vi "SMC_calibrate.vi"(8 "error in (no error)":errorcluster) -> (0 "error out":errorcluster)   [LabVIEW 2015]
uses:
  SMC_SubVIs.llb/SMC_ManagerMode.ctl
  SMC_SubVIs.llb/glb_stop.vi
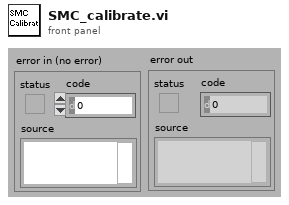
[diagram p1: front panel]
types:
  T1 = typedef "SMC_ManagerMode.ctl" = enum16{"Init", "Get", "SetPosition", "SetStatus", "SetMoving", "SetControllerNr"}
  T2 = typedef "SMC Paras.ctl" = cluster{"VENUS Language":T3, "Number of Axis":u8, "Controller Nr":u8, "Simulation":bool}
  T3 = typedef "VENUSNr.ctl" = enum16{"VENUS 2", "VENUS 1"}
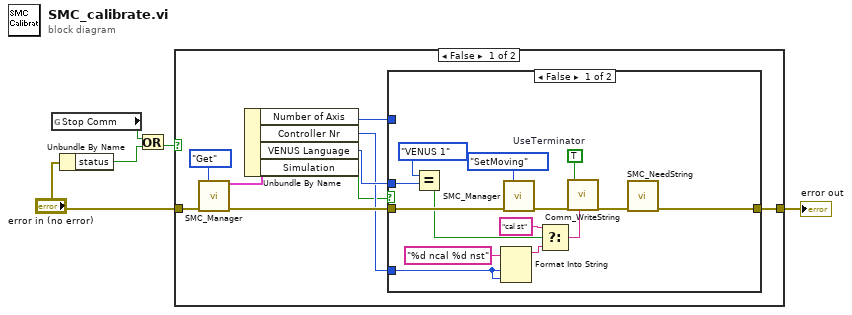
[diagram p0: block diagram]
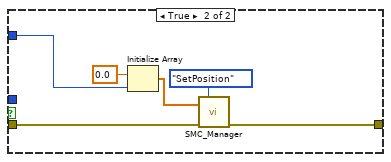
[diagram p2: hidden frame]
diagram:
  n1 = global read "glb_stop.vi" "Stop Comm"() -> (w3:bool)
  n2 = Unbundle By Name("error in (no error)") -> ("status"=w2:bool)
  n3 = Or(x=w3, y=w2) -> (x .or. y?=w1:bool)
  n4 = case shown="False" w1 {
    tunnel: "error in (no error)" -> [w11 w35]
    tunnel: [w14 w35] -> w4
    frame False {
      n5 = call "SMC_Manager.vi"("Mode"=SMC_ManagerMode."Get", "error in (no error)"=w11) -> ("SMC Parameter Out"=w10:T2, "error out"=w12:errorcluster)  [unwired: 9 in, 3 out]
      n6 = Unbundle By Name(w10) -> ("Number of Axis"=w7:u8, "Controller Nr"=w8:u8, "VENUS Language"=w9:T3, "Simulation"=w6:bool)
      n7 = case shown="False" w6 {
        tunnel: w12 -> [w28 w33]
        tunnel: [w25 w32] -> w14
        tunnel: w9 -> [w23 _]
        tunnel: w8 -> [w16 _]
        tunnel: w7 -> [_ w29]
        frame False {
          w15 = TRUE  # UseTerminator
          n8 = Equal?(x=enum16{"VENUS 2", "VENUS 1"}."VENUS 1", y=w23) -> (x = y?=w21:bool)
          n9 = Format Into String(format string="%d ncal %d nst" ("Format String"), w16, w16) -> (resulting string=w18:string)  [unwired: 2 in, 1 out]
          n10 = call "SMC_Manager.vi"("Mode"=SMC_ManagerMode."SetMoving", "error in (no error)"=w28) -> ("error out"=w24:errorcluster)  [unwired: 9 in, 4 out]
          n11 = Select(t="cal st" ("Substring"), s=w21, f=w18) -> (s? t:f=w20:string)
          n12 = call "Comm_WriteString.vi"("string to write"=w20, "error in (no error)"=w24, "UseTerminator"=w15) -> ("error out"=w26:errorcluster)  [unwired: 8 in]
          n13 = call "SMC_NeedString.vi"("error in (no error)"=w26) -> ("error out"=w25:errorcluster)  [unwired: 9 in, 1 out]
        }
        frame True {
          n14 = Initialize Array(0.0 ("Element Data"), w29) -> (w30:dbl[])
          n15 = call "SMC_Manager.vi"("Mode"=SMC_ManagerMode."SetPosition", "PosArraySimu"=w30, "error in (no error)"=w33) -> ("error out"=w32:errorcluster)  [unwired: 8 in, 4 out]
        }
      }
    }
    frame True {
      # "Error, do nothing"
    }
  }
  "error out" <- w4
